vi "Adaptive Noise Cancellation (FPGA).vi"() -> ()   [LabVIEW 2014]
doc: "This VI runs on an FPGA target. This VI acquires signals, applies an LMS adaptive filter to the signals, and sends the signals before and after ANC back to the host via DMA. This VI calls the FXP LMS VI to perform fixed-point adaptive filtering. Use the IP Generator to generate the FXP LMS VI. If you need different fixed-point settings for the FXP LMS VI, use the IP Generator to re-generate the FXP LMS VI. \n\nAfter you edit this VI or change the configuration of the FPGA target, you need to re-compile this VI."
uses:
  <vilib>/LabVIEW Targets/FPGA/cRIO/shared/nicrio_ModuleControls/nicrio_cRIO-9233_DataRatesRing.ctl
  <vilib>/rvi/eio/common/nirviEmuTemplateMethod_errors.vi
  <vilib>/rvi/eio/common/nirviEmuTemplatePropertySet_noerrors.vi
  <vilib>/rvi/Emulation/niFpgaGetClockAttributes.vi
  <vilib>/rvi/Emulation/niFpgaSctlEmulationGetInTimedLoop.vi
  <vilib>/rvi/Emulation/niFpgaEmulationReportErrorSimple.vi
  <vilib>/rvi/Emulation/niFpgaCriticalErrorInLSC.vi
  <vilib>/rvi/interface/RandomDataEmulation/niFpgaRandomDataHandleErrors.vi
  <vilib>/eio/EIONode/EIONode.xnode
  <vilib>/eio/EIOPropertyNode/EIOPropertyNode.xnode
  <vilib>/rvi/DataTransferAndStorage/Container/XNode/niFpgaContainer.xnode
  <vilib>/rvi/interface/RandomDataEmulation/nirviRandomDataFpgaReadWriteTemplate.vi
  <vilib>/rvi/eio/common/nirviEmuTemplatePropertyGet_errors.vi
  <vilib>/rvi/eio/common/nirviEmuTemplatePropertyGet_noerrors.vi
  <vilib>/rvi/eio/common/nirviEmuTemplatePropertySet_errors.vi
panel:
  in  "start":bool
  in  "stop":bool
  in  "step size":fxp<+/-,16,-1>=0.01000213623046875
  in  "reset? (F)":bool
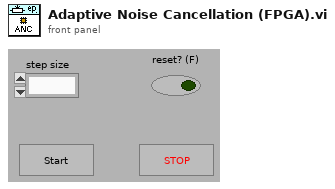
[diagram p1: front panel]
types:
  T1 = typedef "nicrio_cRIO-9233_DataRatesRing.ctl" = u8
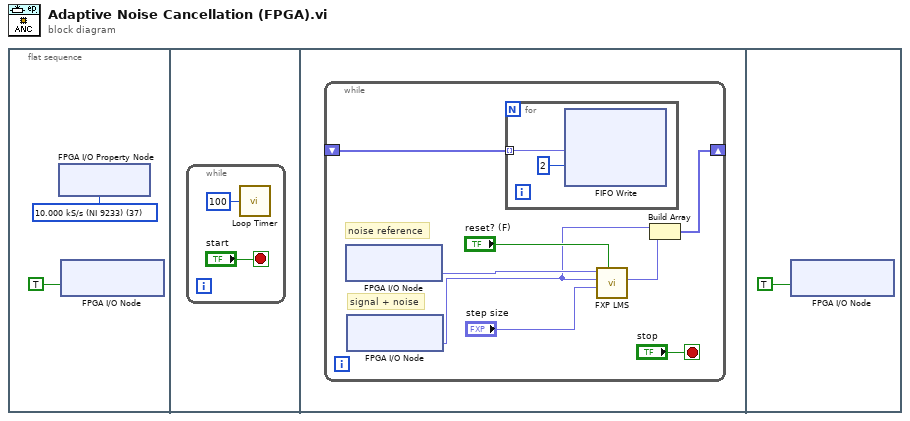
[diagram p0: block diagram]
diagram:
  n1 = flat-sequence {
    frame #0 {
      w1 = T1 37 items=["50.000 kS/s (NI 9233)"=2, "33.333 kS/s (NI 9233)"=3, "25.000 kS/s (NI 9233)"=34, "16.667 kS/s (NI 9233)"=35, "12.500 kS/s (NI 9233)"=36, "10.000 kS/s (NI 9233)"=37, "  8.333 kS/s (NI 9233)"=38, "  7.143 kS/s (NI 9233)"=39, "  6.250 kS/s (NI 9233)"=40, "  5.556 kS/s (NI 9233)"=41, "  5.000 kS/s (NI 9233)"=42, "  4.545 kS/s (NI 9233)"=43, "  4.167 kS/s (NI 9233)"=44, "  3.846 kS/s (NI 9233)"=45, "  3.571 kS/s (NI 9233)"=46, "  3.333 kS/s (NI 9233)"=47, "  3.125 kS/s (NI 9233)"=48, "  2.941 kS/s (NI 9233)"=49, "  2.778 kS/s (NI 9233)"=50, "  2.632 kS/s (NI 9233)"=51, "  2.500 kS/s (NI 9233)"=52, "  2.381 kS/s (NI 9233)"=53, "  2.273 kS/s (NI 9233)"=54, "  2.174 kS/s (NI 9233)"=55, "  2.083 kS/s (NI 9233)"=56, "  2.000 kS/s (NI 9233)"=57] ("Data Rate")
      n2 = xnode "FPGA I/O Property Node"("Data Rate"=w1) -> ()  [unwired: 1 in, 1 out]
      n3 = xnode "FPGA I/O Node"("Mod1/Start"=TRUE ("Start")) -> ()  [unwired: 1 in, 1 out]
    }
    frame #1 {
      n4 = while {
        stop <- "start" stop-if-true
        n5 = call "Loop Timer"("Count(Ticks)"=u32 100) -> ()  [unwired: 1 out]
      }
    }
    frame #2 {
      n6 = while {
        shift-right: [w10] -> _
        shift-left: _ -> [w8]
        stop <- "stop" stop-if-true
        # "signal + noise"
        # "noise reference"
        n7 = xnode "FPGA I/O Node"() -> ("Mod1/AI0"=w6:fxp<+/-,24,4>)  [unwired: 1 in, 1 out]
        n8 = xnode "FPGA I/O Node"() -> ("Mod1/AI1"=w5:fxp<+/-,24,4>)  [unwired: 1 in, 1 out]
        n9 = for {
          tunnel: w8 -> [w14] mode=indexing
          n10 = xnode ("FIFO Write")("Element"=w14, "Timeout"=2) -> ()  [unwired: 1 in, 2 out]
        }
        n11 = call "FXP LMS.vi"("reset? (F)"="reset? (F)", "step size"="step size", "d(n)"=w5, "x(n)"=w6) -> ("e(n)"=w7:fxp<+/-,24,4>)  [unwired: 7 out]
        n12 = Build Array(w5, w7) -> (w10:fxp<+/-,24,4>[])
      }
    }
    frame #3 {
      n13 = xnode "FPGA I/O Node"("Mod1/Stop"=TRUE ("Stop")) -> ()  [unwired: 1 in, 1 out]
    }
  }
